vi "IMAQ FPGA CXP Pixel Buffer 8-Bit x 32.vi"(7 "Reset":bool, 8 "Read":bool, 9 "Tap":u8=8, 10 "Valid Bytes":u8, 11 "Pixel Data In U8x32":u8[](array[numeric])=[0, 0, 0, 0, 0, 0, 0, 0, 0, 0, 0, 0, 0, 0, 0, 0, 0, 0, 0, 0, 0, 0, 0, 0, 0, 0, 0, 0, 0, 0, 0, 0]) -> (2 "#Elements Read":u8, 3 "Pixel Data Out U8x8":u8[](array[numeric]))   [LabVIEW 2020]
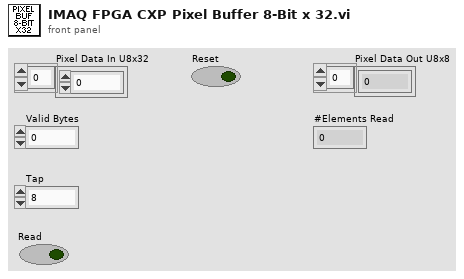
[diagram p1: front panel]
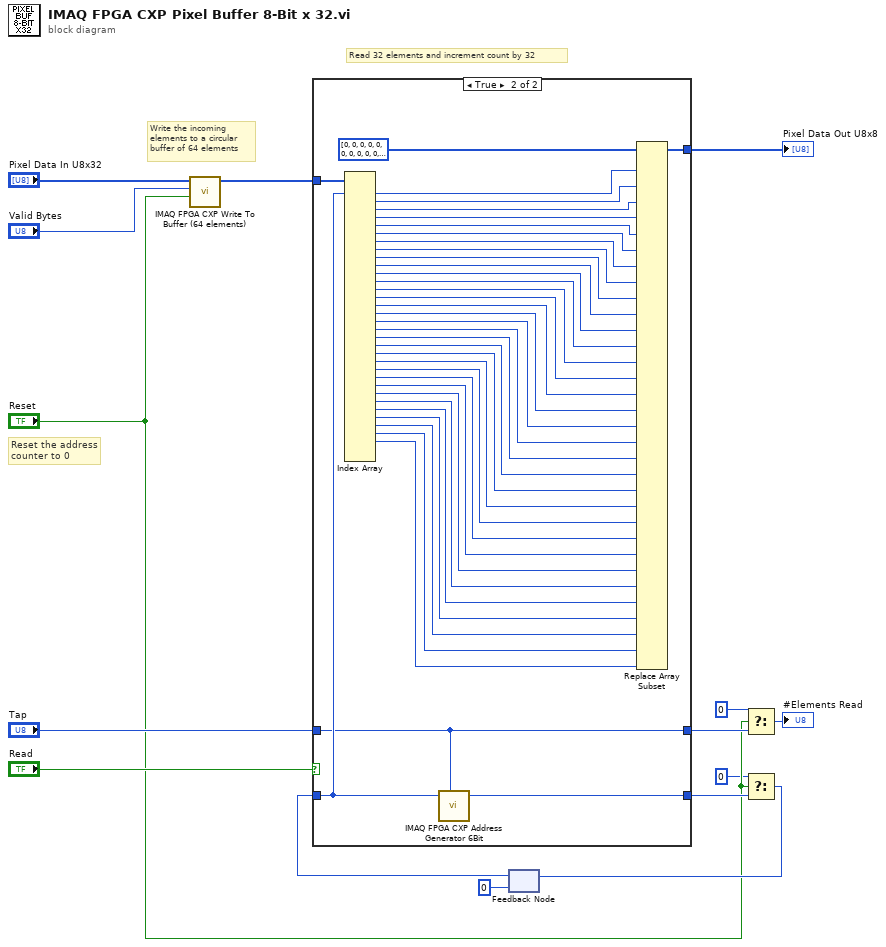
[diagram p0: block diagram]
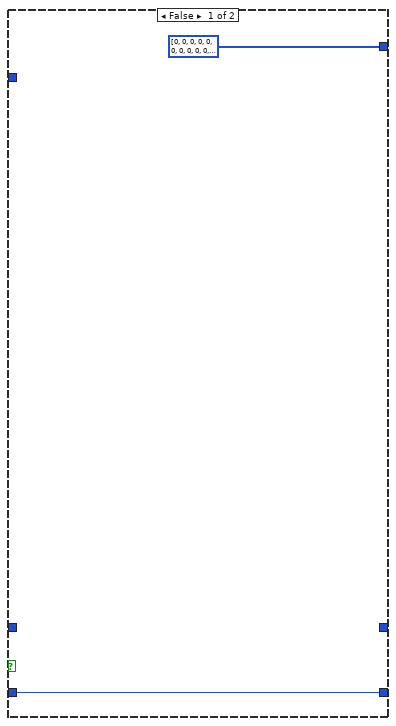
[diagram p2: hidden frame]
diagram:
  # "Reset the address\ncounter to 0"
  # "Write the incoming\nelements to a circular\nbuffer of 64 elements"
  # "Read 32 elements and increment count by 32"
  n1 = call <vilib>:"IMAQ FPGA CXP Write To Buffer (64 elements).vi"("Reset"="Reset", "Valid Bytes"="Valid Bytes", "Pixel Data In U8x32"="Pixel Data In U8x32") -> ("Buffer Out"=w9:u8[])  [unwired: 8 in]
  n2 = feedback #1(u8 0 ("y")) -> (w15:u8)
  n3 = case shown="True" "Read" {
    tunnel: w9 -> [_ w55]
    tunnel: [_ w43] -> w5
    tunnel: [u8[] [0, 0, 0, 0, 0, 0, 0, 0, 0, 0, 0, 0, 0, 0, 0, 0, 0, 0, 0, 0, 0, 0, 0, 0, 0, 0, 0, 0, 0, 0, 0, 0] w53] -> w14
    tunnel: [w17 w42] -> w7
    tunnel: w15 -> [w17 w44]
    tunnel: "Tap" -> [_ w43]
    frame False {
    }
    frame True {
      n4 = Index Array(array=w55, index #1=w44) -> (element #1=w52:u8, element #2=w51:u8, element #3=w50:u8, element #4=w49:u8, element #5=w48:u8, element #6=w47:u8, element #7=w46:u8, element #8=w45:u8, element #9=w41:u8, element #10=w40:u8, element #11=w39:u8, element #12=w38:u8, element #13=w37:u8, element #14=w36:u8, element #15=w35:u8, element #16=w34:u8, element #17=w18:u8, element #18=w33:u8, element #19=w32:u8, element #20=w31:u8, element #21=w30:u8, element #22=w29:u8, element #23=w28:u8, element #24=w27:u8, element #25=w26:u8, element #26=w25:u8, element #27=w24:u8, element #28=w23:u8, element #29=w22:u8, element #30=w21:u8, element #31=w20:u8, element #32=w19:u8)  [unwired: 33 in, 2 out]
      n5 = call <vilib>:"IMAQ FPGA CXP Address Generator 6Bit.vi"("Base Address"=w44, "Index"=w43) -> ("Address Out"=w42:u8)  [unwired: 7 in]
      n6 = Replace Array Subset(array=u8[] [0, 0, 0, 0, 0, 0, 0, 0, 0, 0, 0, 0, 0, 0, 0, 0, 0, 0, 0, 0, 0, 0, 0, 0, 0, 0, 0, 0, 0, 0, 0, 0], new element #1=w52, new element #2=w51, new element #3=w50, new element #4=w49, new element #5=w48, new element #6=w47, new element #7=w46, new element #8=w45, new element #9=w41, new element #10=w40, new element #11=w39, new element #12=w38, new element #13=w37, new element #14=w36, new element #15=w35, new element #16=w34, new element #17=w18, new element #18=w33, new element #19=w32, new element #20=w31, new element #21=w30, new element #22=w29, new element #23=w28, new element #24=w27, new element #25=w26, new element #26=w25, new element #27=w24, new element #28=w23, new element #29=w22, new element #30=w21, new element #31=w20, new element #32=w19) -> (w53:u8[])  [unwired: 32 in]
    }
  }
  "Pixel Data Out U8x8" <- w14
  n7 = Select(t=u8 0 ("Tap"), s="Reset", f=w5) -> (s? t:f=→"#Elements Read":u8)
  n8 = Select(t=u8 0 ("y"), s="Reset", f=w7) -> (s? t:f=w8:u8)
  n9 = feedback-in #1(w8) -> ()
